vi "Case structure Numeric.vi"() -> ()   [LabVIEW 2020]
panel:
  in  "Numeric":dbl
  # "Case structure Numeric"
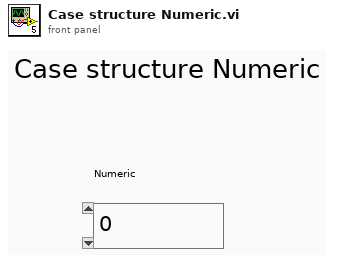
[diagram p1: front panel]
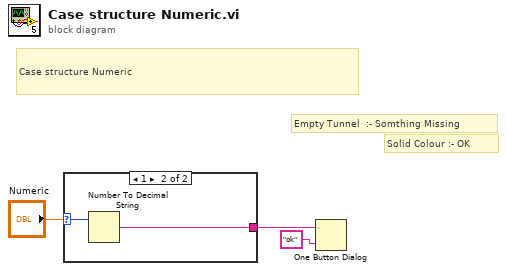
[diagram p0: block diagram]
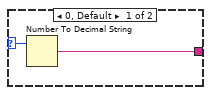
[diagram p2: hidden frame]
diagram:
  # "Solid Colour :- OK"
  # "Empty Tunnel  :- Somthing Missing"
  # "Case structure Numeric"
  n1 = case shown="1" "Numeric" {
    selector: "Numeric" -> [w5 w7]
    tunnel: [w4 w6] -> w2
    frame 0, Default {
      n2 = Number To Decimal String(number=w5) -> (decimal integer string=w4:string)  [unwired: 1 in]
    }
    frame 1 {
      n3 = Number To Decimal String(number=w7) -> (decimal integer string=w6:string)  [unwired: 1 in]
    }
  }
  n4 = One Button Dialog(message=w2, button name ("OK")="ok") -> ()  [unwired: 1 out]
